vi "Main FPGA.vi"() -> ()   [LabVIEW 2014]
uses:
  <vilib>/rvi/Emulation/niFpgaGetClockAttributes.vi
  <vilib>/rvi/Emulation/niFpgaSctlEmulationGetInTimedLoop.vi
  <vilib>/rvi/Emulation/niFpgaEmulationReportErrorSimple.vi
  <vilib>/rvi/eio/common/nirviEmuTemplateMethod_errors.vi
  <vilib>/rvi/Emulation/niFpgaCriticalErrorInLSC.vi
  <vilib>/rvi/Emulation/niFpgaProcessEmulError.vi
  <vilib>/eio/EIONode/EIONode.xnode
panel:
  in  "SAFETY ON":bool
  out "STOP ??":bool
  out "System Reset":bool
  out "Czas od ostatniego sygnalu":u64
  in  "watchdog":bool
  in  "dozwolony czas pomiedzy watchdogiem":u64=5000
  in  "wlacz watchdoga":bool
  in  "RESET STM":bool
  out "temperatura":sgl
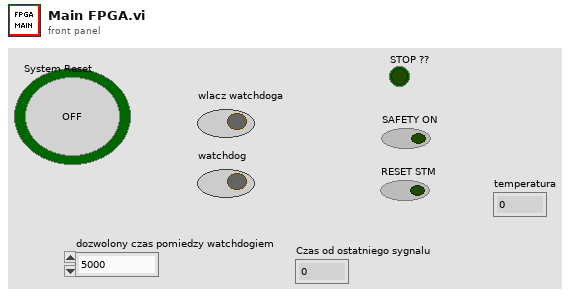
[diagram p1: front panel]
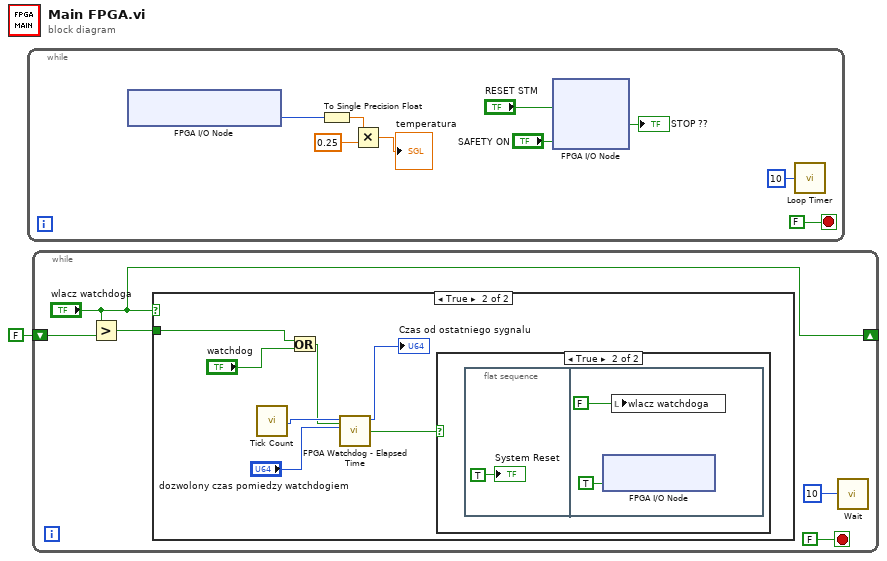
[diagram p0: block diagram]
diagram:
  n1 = while {
    stop <- FALSE stop-if-true
    n2 = xnode "FPGA I/O Node"() -> ("Chassis Temperature"=w6:i16)  [unwired: 1 in, 1 out]
    n3 = To Single Precision Float(number=w6) -> (single precision float=w8:sgl)
    n4 = Multiply(x=w8, y=sgl 0.25) -> (x*y=→"temperatura":sgl)
    n5 = xnode "FPGA I/O Node"("DIO4"="RESET STM", "DIO6"="SAFETY ON") -> ("DIO5"=→"STOP ??":bool)  [unwired: 3 in, 3 out]
    n6 = call "Loop Timer"("Count(uSec)"=u32 10) -> ()  [unwired: 1 out]
  }
  n7 = while {
    shift-right: ["wlacz watchdoga"] -> _
    shift-left: FALSE -> [w12]
    stop <- FALSE stop-if-true
    n8 = Greater?(x="wlacz watchdoga", y=w12) -> (0:w13:bool)
    n9 = case shown="True" "wlacz watchdoga" {
      tunnel: w13 -> [_ w22]
      frame False {
      }
      frame True {
        n10 = call "Tick Count"() -> ("Tick Count(mSec)"=w19:u32)
        n11 = Or(x=w22, y="watchdog") -> (x .or. y?=w18:bool)
        n12 = call "FPGA Watchdog - Elapsed Time.vi"("Reset"=w18, "Timeout Period"="dozwolony czas pomiedzy watchdogiem", "Current Time"=w19) -> ("Timeout"=w16:bool, "Elapsed Time"=→"Czas od ostatniego sygnalu":u64)  [unwired: 7 in]
        n13 = case shown="True" w16 {
          frame False {
          }
          frame True {
            n14 = flat-sequence {
              frame #0 {
                "System Reset" <- TRUE ("System Reset")
              }
              frame #1 {
                n15 = xnode "FPGA I/O Node"("System Reset"=TRUE) -> ()  [unwired: 1 in, 1 out]
                n16 = local write "wlacz watchdoga"(FALSE ("System Reset")) -> ()
              }
            }
          }
        }
      }
    }
    n17 = call "Wait"("Count(uSec)"=u32 10) -> ()  [unwired: 1 out]
  }
